vi "Read HV Enable Button.vi"(4 "error in":errorcluster) -> (0 "error out":errorcluster, 2 "HV Enable Pressed?":bool)   [LabVIEW 2015]
uses:
  <vilib>/DAQmx/read.llb/DAQmx Read (Digital Bool 1Line 1Point).vi
  <vilib>/DAQmx/miscellaneous.llb/DAQmx Fill In Error Info.vi
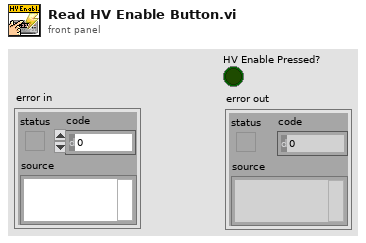
[diagram p1: front panel]
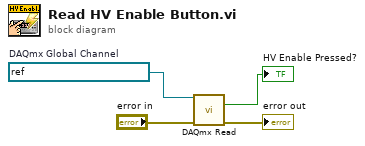
[diagram p0: block diagram]
diagram:
  w4 = refnum<k21> "DI2 HV Enable Button"  # DAQmx Global Channel
  n1 = call-poly <vilib>:"DAQmx Read.vi"("task/channels in"=w4, "error in"="error in") -> ("data"=→"HV Enable Pressed?":bool, "error out"=→"error out":errorcluster)  [unwired: 11 in, 1 out]
